vi "Add Access Log.vi"(8 "error in (no error)":errorcluster, 9 "Response":refnum<class "Response.lvclass">, 10 "Request":refnum<class "Request.lvclass">, 11 "Server in":refnum<class "Server.lvclass">) -> (0 "error out":errorcluster, 3 "Server out":refnum<class "Server.lvclass">)   [LabVIEW 2020, in "HTTP Server.lvlib" / "Server.lvclass"]
uses:
  Server.lvclass
  Server.lvclass/Server.ctl
  lv-http-util/HTTP Utils/Request/Request.lvclass
  Access Log Entry.ctl
  lv-http-util/HTTP Utils/Response/Response.lvclass
  lv-uri/URI/URI/URI.lvclass
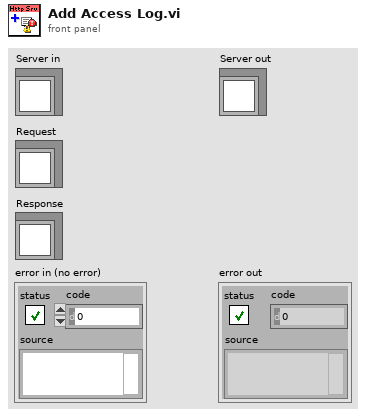
[diagram p1: front panel]
types:
  T1 = typedef "HTTP Server.lvlib/Server.lvclass/Access Log Entry.ctl" = cluster{"Time Stamp":timestamp, "Client":string, "Code":u16, "Info":string}
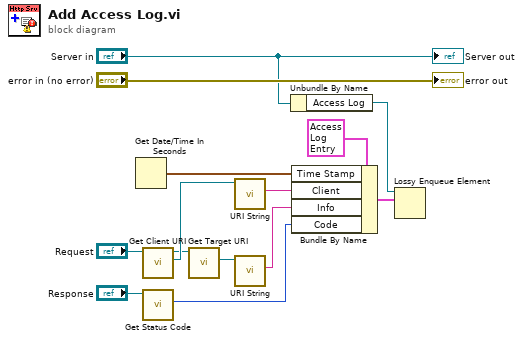
[diagram p0: block diagram]
diagram:
  n1 = Get Date/Time In Seconds() -> (seconds since 1Jan1904=w11:timestamp)
  n2 = call "Get Client URI.vi"("Request in"="Request") -> ("Client URI"=w10:refnum<class "URI.lvclass">, "Request out"=w6:refnum<class "Request.lvclass">)  [unwired: 8 in, 1 out]
  n3 = call "Get Status Code.vi"("Response in"="Response") -> ("Status Code"=w7:u16)  [unwired: 8 in, 2 out]
  n4 = call "Get Target URI.vi"("Request in"=w6) -> ("Target URI"=w5:refnum<class "URI.lvclass">)  [unwired: 8 in, 2 out]
  n5 = call "URI String.vi"("URI in"=w10) -> ("URI String"=w9:string)  [unwired: 9 in, 1 out]
  n6 = call "URI String.vi"("URI in"=w5) -> ("URI String"=w4:string)  [unwired: 9 in, 1 out]
  n7 = Unbundle By Name("Server in") -> ("Access Log"=w2:refnum<queue>)
  n8 = Bundle By Name(cluster=T1 {"Time Stamp"=timestamp(0 s since 1904-01-01), "Client"="", "Code"=0, "Info"=""} ("Log Entry"), "Time Stamp"=w11, "Client"=w9, "Info"=w4, "Code"=w7) -> (w1:T1)
  n9 = Lossy Enqueue Element(queue=w2, element=w1) -> ()  [unwired: 1 in, 4 out]
  "error out" <- "error in (no error)"
  "Server out" <- "Server in"
